vi "校准任务设置.vi"(11 "用户事件":refnum<user-event>) -> ()   [LabVIEW 2016, in "斯坦道CODMn新电路板.lvlib"]
panel:
  in  "校准任务存档":T1[](array[typedef])
  out "字符串":string
  out "校准运行状态":bool
  in  "校准任务":T1[](array[typedef])
  in  "停止":bool
  in  "设置":bool
  in  "执行":bool
  in  "删除":bool
  in  "清空":bool
  in  "任务列表":i32(listbox)
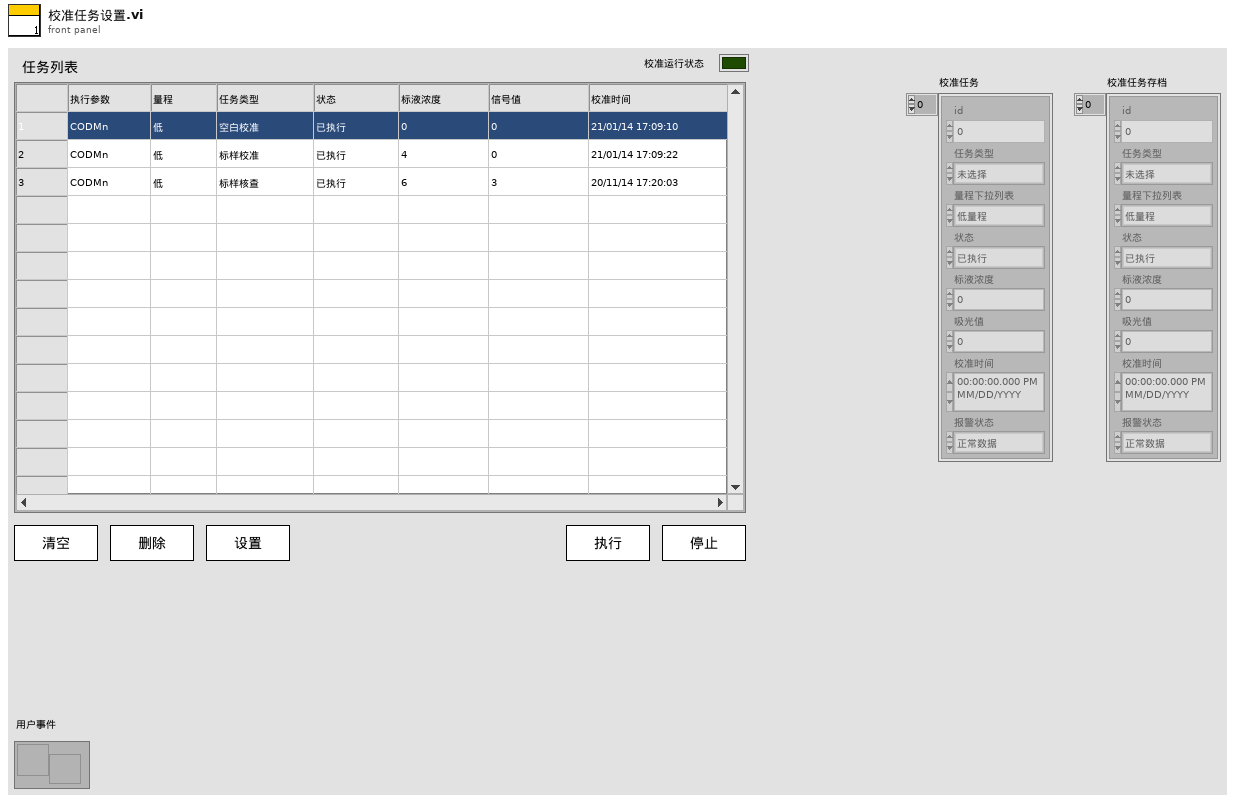
[diagram p1: front panel]
types:
  T1 = typedef "校准任务.ctl" = cluster{"id":u16, "任务类型":enum16{"未选择", "空白校准", "标样校准", "标样核查", "零点核查", "跨度核查"}, "量程下拉列表":enum16{"低量程", "高量程"}, "状态":enum16{"已执行", "待执行", "执行中", "停止"}, "标液浓度":dbl, "吸光值":dbl, "校准时间":timestamp, "报警状态":enum16{"正常数据", "报警数据"}}
  T2 = cluster{"校准类型":string, "校准数据":cluster{"时间":timestamp, "标液值":dbl, "检测值":dbl, "吸光值":dbl}}
  T3 = enum8{"Enabled", "Disabled", "Disabled and Grayed Out"}
  T4 = typedef "LVPoint32TypeDef.ctl" = cluster{"Horizontal":i32, "Vertical":i32}
  T5 = typedef "LVRowAndColumnTypeDef.ctl" = cluster{"Row":i32, "Column":i32}
  T6 = enum16{"未选择", "空白校准", "标样校准", "标样核查", "零点核查", "跨度核查"}
  T7 = cluster{"id":u16, "任务类型":enum16{"未选择", "空白校准", "标样校准", "标样核查", "零点核查", "跨度核查"}, "量程下拉列表":enum16{"低量程", "高量程"}, "状态":enum16{"已执行", "待执行", "执行中", "停止"}, "标液浓度":dbl, "吸光值":dbl, "校准时间":timestamp, "报警状态":enum16{"正常数据", "报警数据"}}
  T8 = enum32{"Bad", "Idle", "Run top level", "Running"}
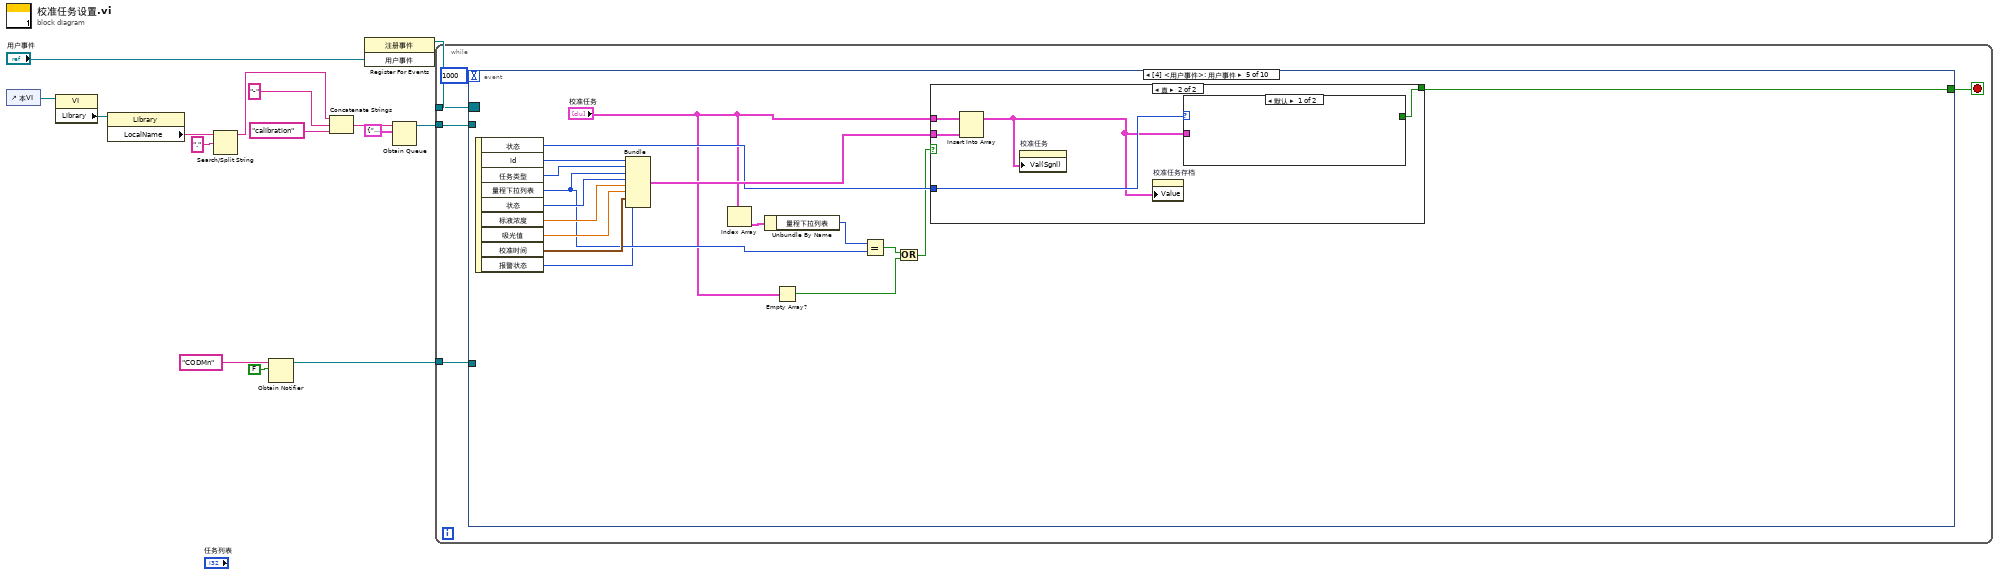
[diagram p0: block diagram]
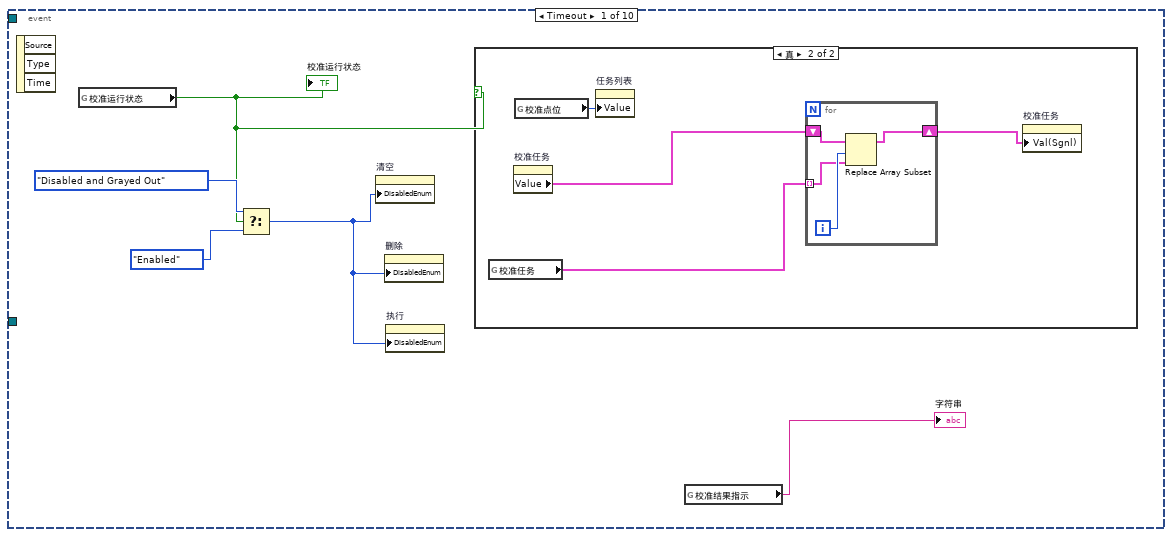
[diagram p2: hidden frame]
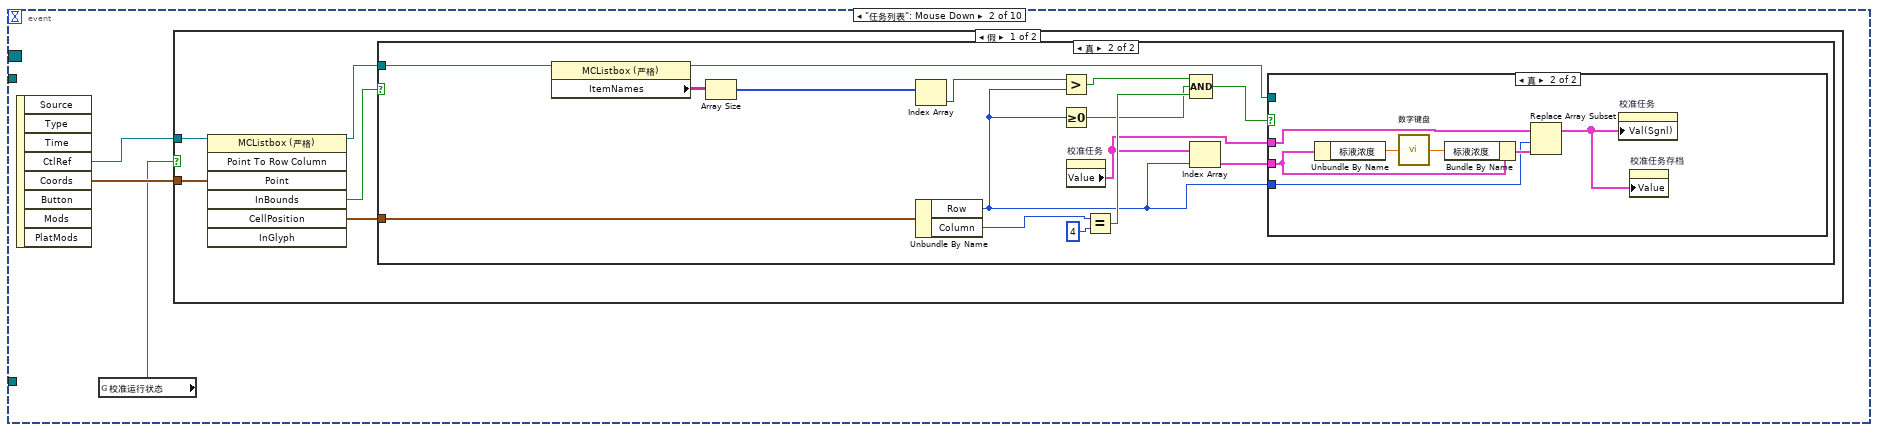
[diagram p4: hidden frame]
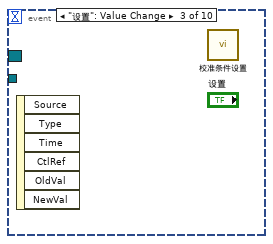
[diagram p8: hidden frame]
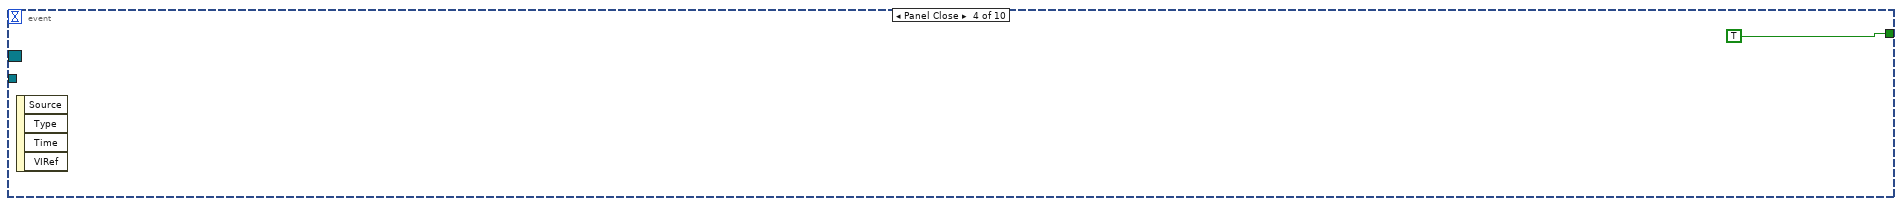
[diagram p9: hidden frame]
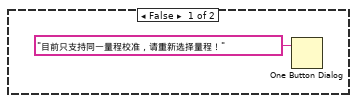
[diagram p10: hidden frame]
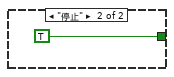
[diagram p11: hidden frame]
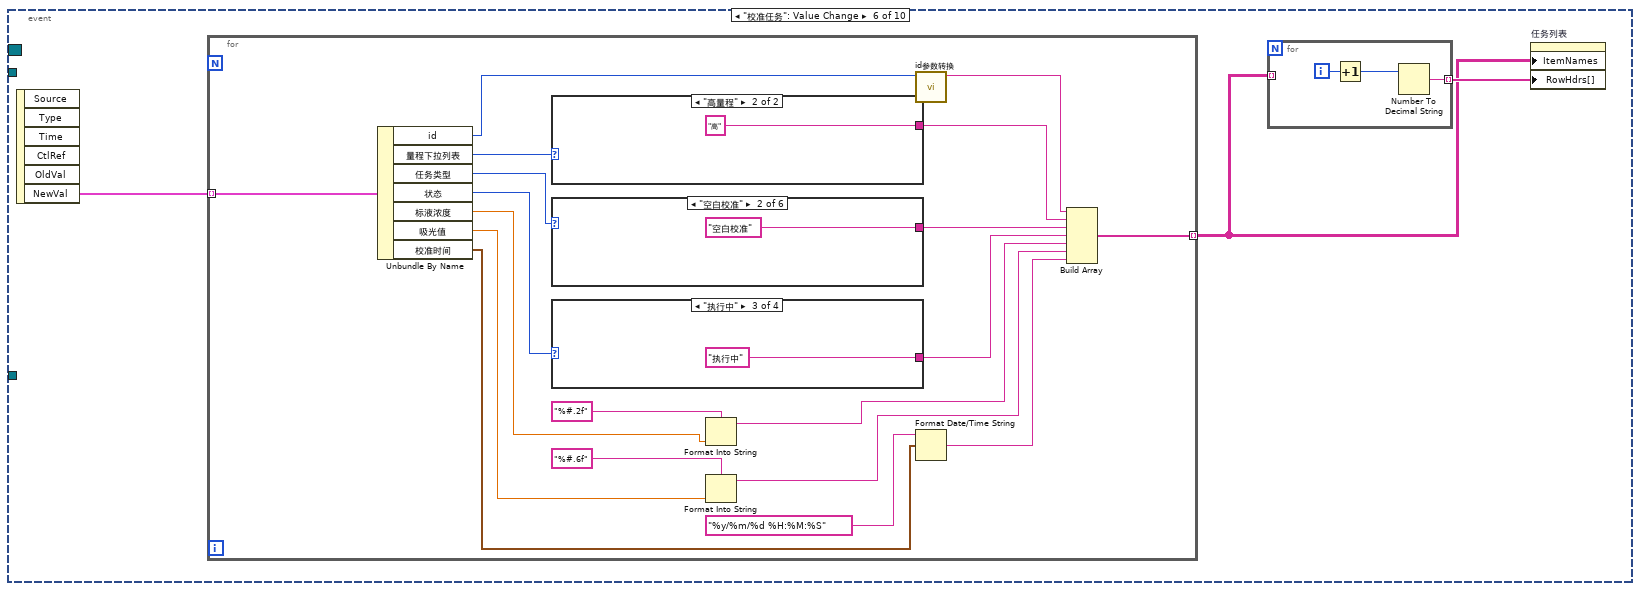
[diagram p12: hidden frame]
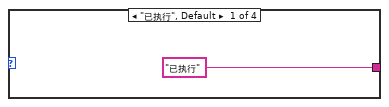
[diagram p13: hidden frame]
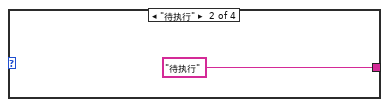
[diagram p14: hidden frame]
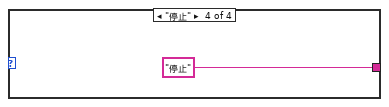
[diagram p15: hidden frame]
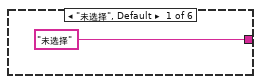
[diagram p16: hidden frame]
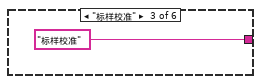
[diagram p17: hidden frame]
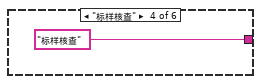
[diagram p18: hidden frame]
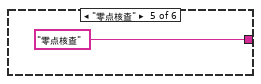
[diagram p19: hidden frame]
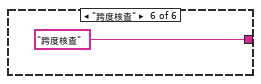
[diagram p20: hidden frame]
diagram:
  n1 = control-ref of="本VI"() -> (w14:refnum<vi>)
  n2 = property class="VI"(reference=w14) -> ("Library"=w15:refnum<vi>)  [unwired: 1 in, 2 out]
  n3 = property class="Library"(reference=w15) -> ("LocalName"=w13:string)  [unwired: 1 in, 2 out]
  n4 = Search/Split String(string=w13, search string/char (-)="." ("搜索字符串/字符(-)")) -> (substring before match=w11:string)  [unwired: 1 in, 2 out]
  n5 = Obtain Notifier(name (unnamed)="CODMn" ("字符串"), notification data type=FALSE) -> (notifier out=w2:refnum<notifier>)  [unwired: 2 in, 2 out]
  n6 = Concatenate Strings(w11, "-" ("字符串"), "calibration" ("名称或相对路径")) -> (w8:string)
  n7 = register-events("用户事件") -> (reference out=w5:refnum<event-registration>)  [unwired: 2 in, 1 out]
  n8 = Obtain Queue(name (unnamed)=w8, element data type=T2 {"校准类型"="", "校准数据"={"时间"=timestamp(0 s since 1904-01-01), "标液值"=0.0, "检测值"=0.0, "吸光值"=0.0}}) -> (queue out=w6:refnum<queue>)  [unwired: 3 in, 2 out]
  n9 = while {
    tunnel: w6 -> [w19]
    tunnel: w5 -> [w18]
    tunnel: w2 -> [w17]
    stop <- w20 stop-if-true
    n10 = event shown="[4] <用户事件>: 用户事件" {
      selector: w18 -> [_ _ _ _ _ _ _ _ _ _]
      dyn-events: _ -> [_ _ _ _ _ _ _ _ _ _]
      timeout: 1000 -> [_ _ _ _ _ _ _ _ _ _]
      tunnel: [_ _ _ TRUE w81 _ _ _ _ _] -> w20
      tunnel: w19 -> [_ _ _ _ _ _ _ _ _ _]
      tunnel: w17 -> [_ _ _ _ _ _ _ _ _ w147]
      event Timeout {
        n11 = event-data() -> ()  [unwired: 1 in, 3 out]
        n12 = global read "VARCODMn全局变量.vi" "校准运行状态"() -> (w22:bool)
        "校准运行状态" <- w22
        n13 = Select(t=T3."Disabled and Grayed Out" ("禁用"), s=w22, f=T3."Enabled" ("禁用")) -> (s? t:f=w24:T3)
        n14 = property on="清空" class="Bool"("DisabledEnum"=w24) -> ()  [unwired: 2 in, 2 out]
        n15 = property on="删除" class="Bool"("DisabledEnum"=w24) -> ()  [unwired: 2 in, 2 out]
        n16 = property on="执行" class="Bool"("DisabledEnum"=w24) -> ()  [unwired: 2 in, 2 out]
        n17 = case shown="真" w22 {
          frame False {
          }
          frame True {
            n18 = global read "VARCODMn全局变量.vi" "校准任务"() -> (w27:T1[])
            n19 = property on="校准任务" class="Arr (严格)"() -> ("Value"=w28:T1[])  [unwired: 2 in, 2 out]
            n20 = global read "VARCODMn全局变量.vi" "校准点位"() -> (w29:u16)
            n21 = property on="任务列表" class="MCListbox (严格)"("Value"=w29) -> ()  [unwired: 2 in, 2 out]
            n22 = for {
              tunnel: w27 -> [w31] mode=indexing
              shift-right: [w30] -> w26
              shift-left: w28 -> [w33]
              i -> [w32]
              n23 = Replace Array Subset(array=w33, new element=w31, index=w32) -> (w30:T1[])
            }
            n24 = property on="校准任务" class="Arr (严格)"("Val(Sgnl)"=w26) -> ()  [unwired: 2 in, 2 out]
          }
        }
        n25 = global read "VARCODMn全局变量.vi" "校准结果指示"() -> (→"字符串":string)
      }
      event "任务列表": Mouse Down {
        n26 = event-data() -> ("CtlRef"=w36:refnum<vi>, "Coords"=w35:T4)  [unwired: 1 in, 6 out]
        n27 = global read "VARCODMn全局变量.vi" "校准运行状态"() -> (w34:bool)
        n28 = case shown="假" w34 {
          tunnel: w36 -> [w41 _]
          tunnel: w35 -> [w37 _]
          frame False {
            n29 = invoke class="MCListbox (严格)" method="Point To Row Column"(reference=w41, "Point"=w37) -> (reference out=w38:refnum<vi>, "InBounds"=w40:bool, "CellPosition"=w39:T5)  [unwired: 5 in, 4 out]
            n30 = case shown="真" w40 {
              tunnel: w39 -> [_ w56]
              tunnel: w38 -> [_ w55]
              frame False {
              }
              frame True {
                n31 = property class="MCListbox (严格)"(reference=w55) -> (reference out=w54:refnum<vi>, "ItemNames"=w53:string[][])  [unwired: 1 in, 1 out]
                n32 = Array Size(array=w53) -> (size(s)=w52:i32[])
                n33 = Index Array(array=w52) -> (element=w51:i32)  [unwired: 1 in]
                n34 = Unbundle By Name(w56) -> ("Row"=w42:i32, "Column"=w50:i32)
                n35 = Greater?(x=w51, y=w42) -> (0:w46:bool)
                n36 = Greater Or Equal To 0?(x=w42) -> (x >= 0?=w45:bool)
                n37 = property on="校准任务" class="Arr (严格)"() -> ("Value"=w43:T1[])  [unwired: 2 in, 2 out]
                n38 = Equal?(x=w50, y=4) -> (x = y?=w48:bool)
                n39 = Compound Arithmetic op=AND ("复合运算")(w46, w45, w48) -> (w47:bool)
                n40 = Index Array(array=w43, index=w42) -> (element=w44:T1)
                n41 = case shown="真" w47 {
                  tunnel: w54 -> [_ _]
                  tunnel: w44 -> [_ w62]
                  tunnel: w43 -> [_ w60]
                  tunnel: w42 -> [_ w58]
                  frame False {
                  }
                  frame True {
                    n42 = Unbundle By Name(w62) -> ("标液浓度"=w63:dbl)
                    n43 = call "数字键盘.vi"("OldNumber"=w63) -> ("NewNumber"=w61:dbl)
                    n44 = Bundle By Name(cluster=w62, "标液浓度"=w61) -> (w59:T1)
                    n45 = Replace Array Subset(array=w60, new element=w59, index=w58) -> (w57:T1[])
                    n46 = property on="校准任务" class="Arr (严格)"("Val(Sgnl)"=w57) -> ()  [unwired: 2 in, 2 out]
                    n47 = property on="校准任务存档" class="Arr (严格)"("Value"=w57) -> ()  [unwired: 2 in, 2 out]
                  }
                }
              }
            }
          }
          frame True {
          }
        }
      }
      event "设置": Value Change {
        n48 = event-data() -> ()  [unwired: 1 in, 6 out]
        n49 = call "校准条件设置.vi"() -> ()  [unwired: 12 in]
      }
      event Panel Close {
        n50 = event-data() -> ()  [unwired: 1 in, 4 out]
      }
      event User Event {
        n51 = event-data() -> ("状态"=w73:enum16{"已执行", "待执行", "执行中", "停止"}, "id"=w80:u16, "任务类型"=w78:T6, "量程下拉列表"=w70:enum16{"低量程", "高量程"}, "状态"=w77:enum16{"已执行", "待执行", "执行中", "停止"}, "标液浓度"=w76:dbl, "吸光值"=w75:dbl, "校准时间"=w74:timestamp, "报警状态"=w65:enum16{"正常数据", "报警数据"})  [unwired: 1 in]
        n52 = Bundle("id"=w80, "任务类型"=w78, "量程下拉列表"=w70, "状态"=w77, "标液浓度"=w76, "吸光值"=w75, "校准时间"=w74, "报警状态"=w65) -> (w79:T7)  [unwired: 1 in]
        n53 = Index Array(array="校准任务") -> (element=w72:T1)  [unwired: 1 in]
        n54 = Unbundle By Name(w72) -> ("量程下拉列表"=w71:enum16{"低量程", "高量程"})
        n55 = Empty Array?(array="校准任务") -> (empty?=w66:bool)
        n56 = Equal?(x=w71, y=w70) -> (x = y?=w68:bool)
        n57 = Or(x=w68, y=w66) -> (x .or. y?=w67:bool)
        n58 = case shown="真" w67 {
          tunnel: [_ w87] -> w81
          tunnel: w79 -> [_ w86]
          tunnel: w73 -> [_ w85]
          tunnel: "校准任务" -> [_ w84]
          frame False {
            n59 = One Button Dialog(message="目前只支持同一量程校准，请重新选择量程！" ("消息")) -> ()  [unwired: 1 in, 1 out]
          }
          frame True {
            n60 = Insert Into Array(array=w84, new element=w86) -> (w83:T1[])  [unwired: 1 in]
            n61 = property on="校准任务" class="Arr (严格)"("Val(Sgnl)"=w83) -> ()  [unwired: 2 in, 2 out]
            n62 = property on="校准任务存档" class="Arr (严格)"("Value"=w83) -> ()  [unwired: 2 in, 2 out]
            n63 = case shown="默认" w85 {
              tunnel: [_ TRUE] -> w87
              tunnel: w83 -> [_ _]
              frame Default {
              }
              frame "停止" {
              }
            }
          }
        }
      }
      event "校准任务": Value Change {
        n64 = event-data() -> ("NewVal"=w89:T1[])  [unwired: 1 in, 5 out]
        n65 = for {
          tunnel: w89 -> [w110] mode=indexing
          tunnel: [w92] -> w90 mode=indexing
          n66 = Unbundle By Name(w110) -> ("id"=w109:u16, "量程下拉列表"=w108:enum16{"低量程", "高量程"}, "任务类型"=w107:T6, "状态"=w106:enum16{"已执行", "待执行", "执行中", "停止"}, "标液浓度"=w104:dbl, "吸光值"=w102:dbl, "校准时间"=w100:timestamp)
          n67 = case shown="\"高量程\"" w108 {
            tunnel: ["低" "高"] -> w98
            frame "低量程", Default {
            }
            frame "高量程" {
            }
          }
          n68 = case shown="\"空白校准\"" w107 {
            tunnel: ["未选择" "空白校准" "标样校准" "标样核查" "零点核查" "跨度核查"] -> w97
            frame "未选择", Default {
            }
            frame "空白校准" {
            }
            frame "标样校准" {
            }
            frame "标样核查" {
            }
            frame "零点核查" {
            }
            frame "跨度核查" {
            }
          }
          n69 = case shown="\"执行中\"" w106 {
            tunnel: ["已执行" "待执行" "执行中" "停止"] -> w96
            frame "已执行", Default {
            }
            frame "待执行" {
            }
            frame "执行中" {
            }
            frame "停止" {
            }
          }
          n70 = Format Into String(format string="%#.2f" ("格式字符串"), w104) -> (resulting string=w95:string)  [unwired: 2 in, 1 out]
          n71 = Format Into String(format string="%#.6f" ("格式字符串"), w102) -> (resulting string=w94:string)  [unwired: 2 in, 1 out]
          n72 = call "id参数转换.vi"("id"=w109) -> ("table输出"=w99:string)  [unwired: 10 in]
          n73 = Format Date/Time String(time format string (%c)="%y/%m/%d %H:%M:%S" ("时间格式字符串(%c)"), seconds (now)=w100) -> (date/time string=w93:string)  [unwired: 1 in]
          n74 = Build Array(w99, w98, w97, w96, w95, w94, w93) -> (w92:string[])
        }
        n75 = for {
          tunnel: [w123] -> w91 mode=indexing
          tunnel: w90 -> [_] mode=indexing
          i -> [w125]
          n76 = Increment(x=w125) -> (x+1=w124:i32)
          n77 = Number To Decimal String(number=w124) -> (decimal integer string=w123:string)  [unwired: 1 in]
        }
        n78 = property on="任务列表" class="MCListbox (严格)"("ItemNames"=w90, "RowHdrs[]"=w91) -> ()  [unwired: 2 in, 2 out]
      }
      event "清空": Value Change {
        n79 = event-data() -> ()  [unwired: 1 in, 6 out]
        n80 = property on="校准任务" class="Arr (严格)"("Val(Sgnl)"=T1[] [] ("数组")) -> ()  [unwired: 2 in, 2 out]
      }
      event "删除": Value Change {
        n81 = event-data() -> ()  [unwired: 1 in, 6 out]
        n82 = property on="校准任务" class="Arr (严格)"() -> ("Value"=w129:T1[])  [unwired: 2 in, 2 out]
        n83 = property on="任务列表" class="MCListbox (严格)"() -> ("Value"=w127:i32)  [unwired: 2 in, 2 out]
        n84 = Delete From Array(array=w129, index=w127) -> (array with subset deleted=w128:T1[])  [unwired: 1 in, 1 out]
        n85 = property on="校准任务" class="Arr (严格)"("Val(Sgnl)"=w128) -> ()  [unwired: 2 in, 2 out]
      }
      event "执行": Value Change {
        n86 = event-data() -> ()  [unwired: 1 in, 6 out]
        n87 = global read "VARCODMn全局变量.vi" "校准精度"() -> (w130:dbl)
        n88 = vi-ref "斯坦道CODMn新电路板.lvlib:校准任务流程.vi"() -> (w132:refnum<vi>)
        n89 = global read "VARCODMn全局变量.vi" "校准模型"() -> (w131:enum32{"线性", "多项式", "折线"})
        n90 = property class="VI"(reference=w132) -> (reference out=w135:refnum<vi>, "Name"=w133:string, "Exec.State"=w134:T8)  [unwired: 1 in, 1 out]
        n91 = case shown="\"Idle\"" w134 {
          tunnel: w133 -> [_ w145]
          tunnel: w135 -> [_ _]
          tunnel: w131 -> [_ w138]
          tunnel: w130 -> [_ w137]
          frame "Bad", Default {
          }
          frame "Idle" {
            n92 = Open VI Reference(type specifier VI Refnum (for type only)=refnum<vi> refnum, vi path=w145, options=128 ("选项")) -> (vi reference=w143:refnum<vi>, error out=w141:errorcluster)  [unwired: 3 in]
            n93 = call-by-ref "开始异步调用"(reference=w143, error in=w141, "校准任务"="校准任务存档", "精度"=w137, "模型"=w138) -> (reference out=w142:refnum<vi>, error out=w140:errorcluster)  [unwired: 9 in]
            n94 = Close Reference(reference=w142, error in (no error)=w140) -> ()  [unwired: 1 out]
          }
        }
      }
      event "停止": Value Change {
        n95 = event-data() -> ()  [unwired: 1 in, 6 out]
        n96 = Send Notification(notification=TRUE ("通知"), notifier=w147) -> ()  [unwired: 1 in, 2 out]
      }
    }
  }
